vi "Unflatten JSON Message.vi"(11 "Raw Data":string) -> (0 "error out":errorcluster, 1 "Value Type":T1, 2 "JSON Value":string, 3 "ID":string)   [LabVIEW 2020, in "Stream-Simple-Msg.lvlib" / "Message.lvclass"]
uses:
  Message/Message.lvclass
  <vilib>/IlluminatedG/lv-web-crypto/lv-json/JSON/JSON Item Type.ctl
  <vilib>/IlluminatedG/lv-web-crypto/lv-json/JSON/JSON.lvlib
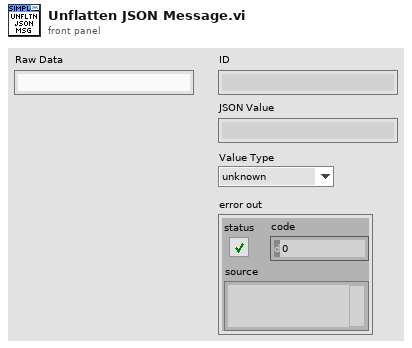
[diagram p1: front panel]
types:
  T1 = typedef "JSON.lvlib/JSON Item Type.ctl" = enum16{"unknown", "null", "Array", "Object", "String", "Number", "Boolean"}
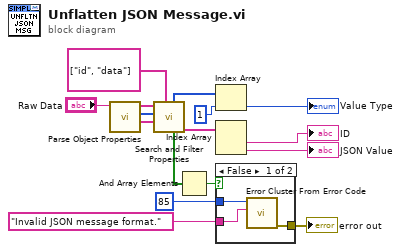
[diagram p0: block diagram]
diagram:
  n1 = call <vilib>:"Parse Object Properties.vi"("JSON String"="Raw Data") -> ("Values"=w13:string[], "Item Types"=w14:T1[], "Keys"=w15:string[])  [unwired: 7 in, 1 out]
  n2 = call <vilib>:"Search and Filter Properties.vi"("Search Keys"=string[] ["id", "data"], "Values In"=w13, "Types In"=w14, "Keys In"=w15) -> ("Filtered Values"=w7:string[], "Item Found"=w5:bool[], "Filtered Types"=w6:T1[])  [unwired: 2 in, 3 out]
  n3 = And Array Elements(Boolean array=w5) -> (logical AND=w4:bool)
  n4 = Index Array(array=w6, index=1) -> (element=→"Value Type":T1)
  n5 = Index Array(array=w7) -> (element #1=→"ID":string, element #2=→"JSON Value":string)  [unwired: 2 in]
  n6 = case shown="False" w4 {
    tunnel: 85 ("error code (0)") -> [w19 _]
    tunnel: "Invalid JSON message format." ("error message (\"\")") -> [w18 _]
    tunnel: [w17 _] -> w1
    frame False {
      n7 = call <vilib>:"Error Cluster From Error Code.vi"("error message (\"\")"=w18, "error code (0)"=w19) -> ("error out"=w17:errorcluster)  [unwired: 7 in]
    }
    frame True {
    }
  }
  "error out" <- w1
